vi "Logging Data.vi"() -> ()   [LabVIEW 2015]
uses:
  Autonomous VIs/Autonomous Commands/Autonomous Command Names.ctl
panel:
  out "Autonomous Play\nRead":bool
  in  "Command Information":T2
  out "Number of Commands":dbl
  out "Play Path":path
  out "Play Name":string
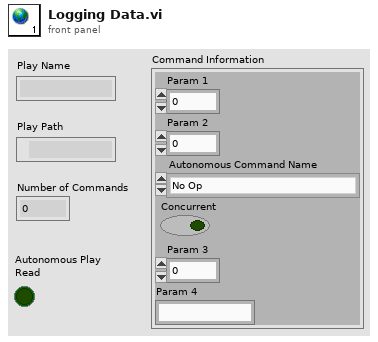
[diagram p1: front panel]
types:
  T1 = typedef "Autonomous Command Names.ctl" = enum16{"No Op", "Drive Time", "Run Motion Profile", "Turn to Heading", "Turn To Target", "Cross Defense", "Fire", "Wait", "Reset Gyro", "Grabber Setpoints", "Manual Grabber", "Roller", "Autorange Command"}
  T2 = cluster{"Param 1":dbl, "Param 2":dbl, "Autonomous Command Name":T1, "Concurrent":bool, "Param 3":dbl, "Param 4":string}
diagram:
